vi "Plot record data.vi"(11 "Array":dbl[][](array[numeric])) -> (2 "Intensity Graph":dbl[][](graph), 3 "All":dbl[][](graph), 4 "Column 4":dbl[](graph), 5 "Column 2":dbl[](graph), 6 "Column 3":dbl[](graph), 7 "Column 1":dbl[](graph))   [LabVIEW 2020]
panel:
  out "min value":dbl
  out "max value":dbl
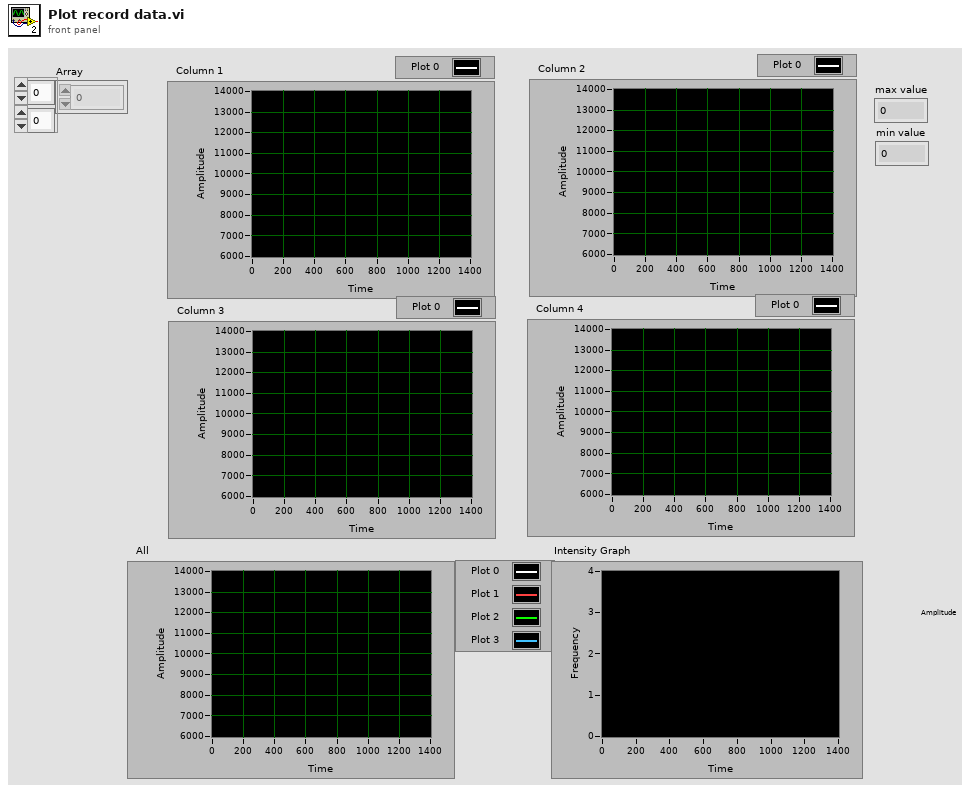
[diagram p1: front panel]
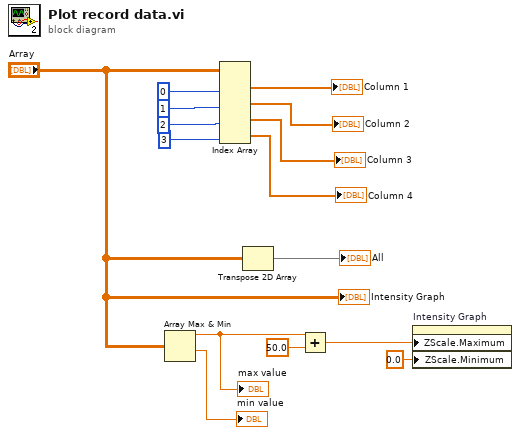
[diagram p0: block diagram]
diagram:
  n1 = Array Max & Min(array="Array") -> (max value=w5:dbl, min value=→"min value":dbl)  [unwired: 2 out]
  "max value" <- w5
  n2 = Index Array(array="Array", index (col) #1=0 ("disabled index (col)"), index (col) #2=1 ("index (col)"), index (col) #3=2 ("index (col)"), index (col) #4=3 ("index (col)")) -> (element #1=→"Column 1":dbl[], element #2=→"Column 2":dbl[], element #3=→"Column 3":dbl[], element #4=→"Column 4":dbl[])  [unwired: 4 in]
  n3 = Transpose 2D Array(2D array="Array") -> (transposed array=→"All":dbl[][])
  n4 = Add(x=w5, y=50.0) -> (x+y=w3:dbl)
  n5 = property on="Intensity Graph" class="IntGraph (strict)"("ZScale.Maximum"=w3, "ZScale.Minimum"=0.0 ("Z Scale.Range:Minimum")) -> ()  [unwired: 2 in, 2 out]
  "Intensity Graph" <- "Array"
